vi "PROXY_display_messages_history.vi"(6 "station_in":T1, 8 "error_in":errorcluster, 9 "All Stations?":bool) -> (0 "error_out":errorcluster)   [LabVIEW 2020]
uses:
  STATION/station.ctl
  FGV/DIAGNOSTICS_message_history_buffer/PROXY_DIAGNOSTICS_message_history_buffer_all_info.ctl
  _misc/DIAGNOSTICS_message_type.ctl
  FGV/DIAGNOSTICS_message_history_display/FGV_PROXY_DIAGNOSTICS_message_history_display.ctl
  FGV/DIAGNOSTICS_message_history_buffer/FGV_PROXY_DIAGNOSTICS_message_history_buffer.ctl
  _misc/AULocalize/SubVIs/RegisterVI.vi
panel:
  in  "clear_messages":bool
  in  "STOP":bool
  in  "station_selector":u16(ring) caption="(ий)Station:" items=["(ий)Station 10", "(ий)Station 20", "(ий)Station 30", "(ий)Station 40", "(ий)Station 50", "(ий)Station 60", "(ий)Station 70", "(ий)Station 80", "(ий)Station 90", "(ий)Station 100", "(ий)Station 110", "(ий)Station 120", "(ий)Station 165", "(ий)ALL"]
  in  "refresh_messages":bool
  in  "messages_history_lbx":i32(listbox)
  # "Message History"
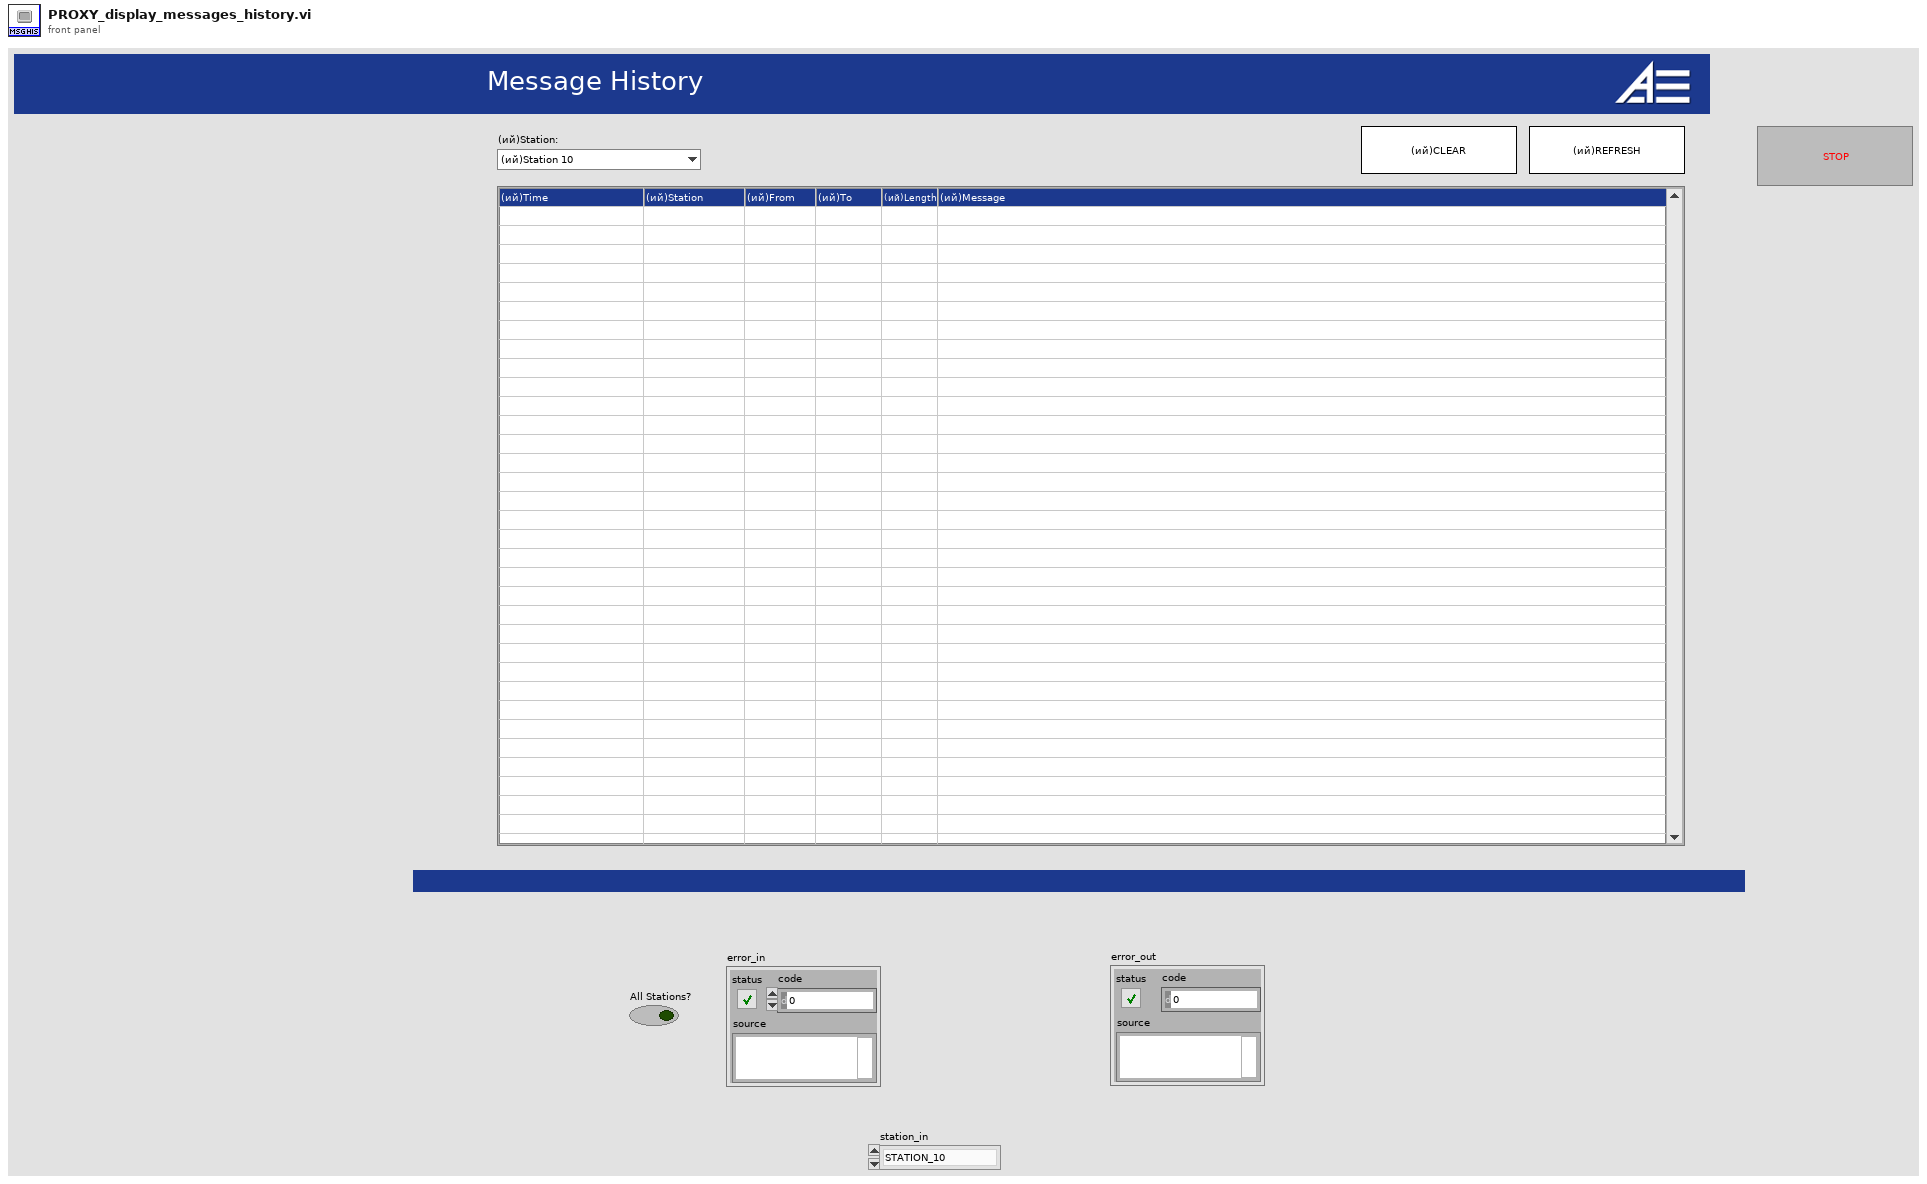
[diagram p1: front panel]
types:
  T1 = typedef "station.ctl" = enum16{"STATION_10", "STATION_20", "STATION_30", "STATION_40", "STATION_50", "STATION_60", "STATION_70", "STATION_80", "STATION_90", "STATION_100", "STATION_110", "STATION_120", "STATION_165", "MAIN"}
  T2 = typedef "FGV_PROXY_DIAGNOSTICS_message_history_display.ctl" = enum16{"initialize", "display_messages"}
  T3 = typedef "PROXY_DIAGNOSTICS_message_history_buffer_all_info.ctl" = cluster{"timestamp":timestamp, "station":T1, "message_type":T4, "message":string, "record":string[]}
  T4 = typedef "DIAGNOSTICS_message_type.ctl" = enum16{"TCP", "SQL"}
  T5 = typedef "FGV_PROXY_DIAGNOSTICS_message_history_buffer.ctl" = enum16{"initialize", "add_TCP_PLC_to_PC", "add_TCP_PC_to_PLC", "add_SQL_PC_to_DB", "add_SQL_transaction", "add_SQL_DB_to_PC", "get_station", "get_all", "clear_station", "clear_all", "save_log"}
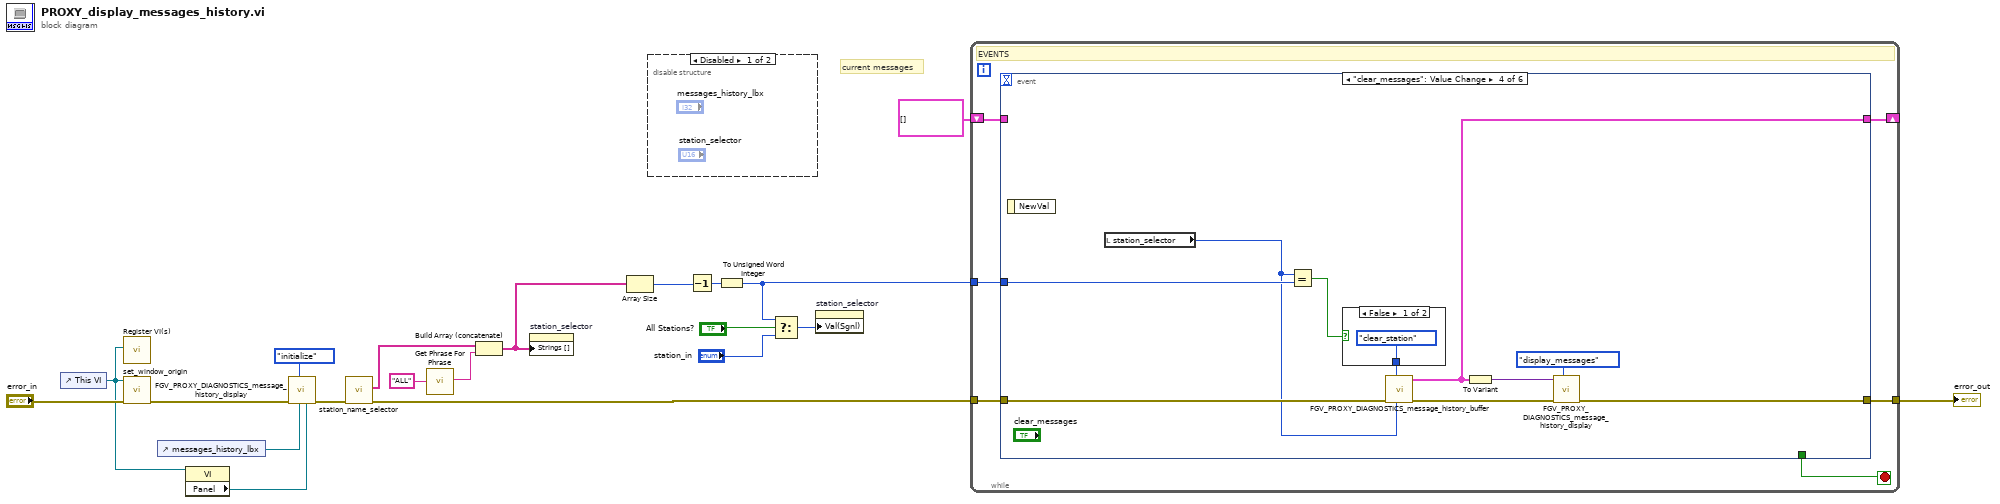
[diagram p0: block diagram]
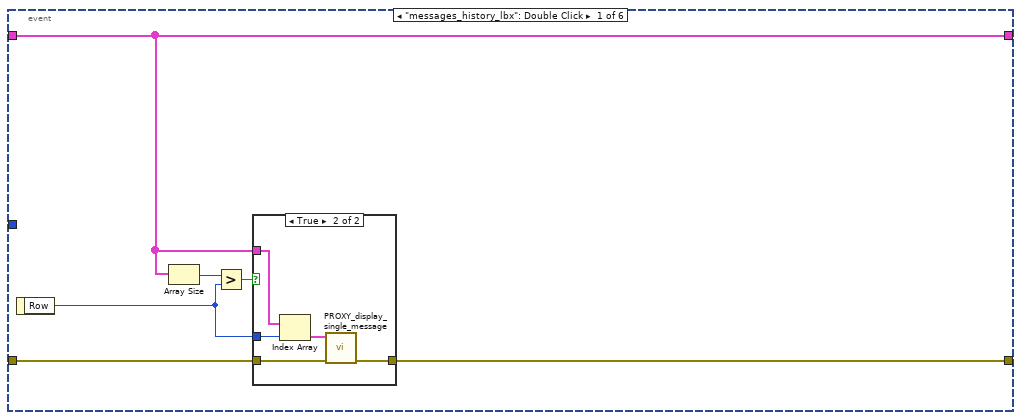
[diagram p3: hidden frame]
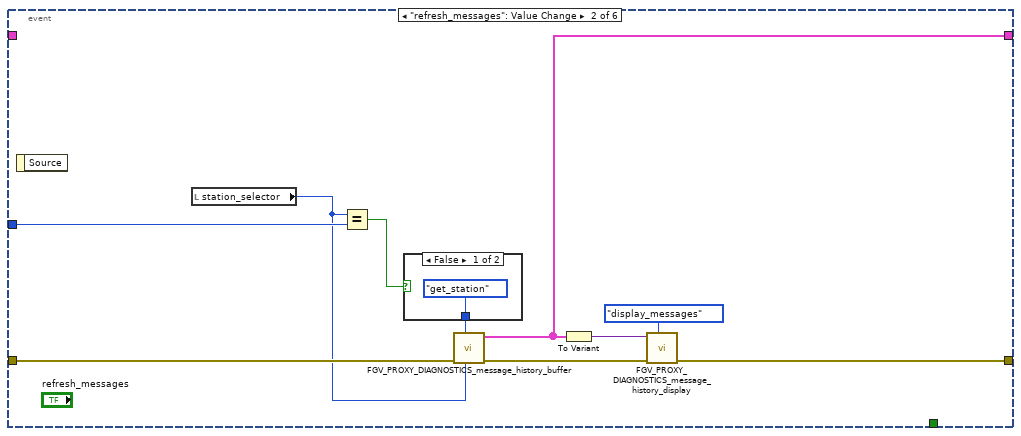
[diagram p5: hidden frame]
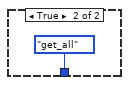
[diagram p6: hidden frame]
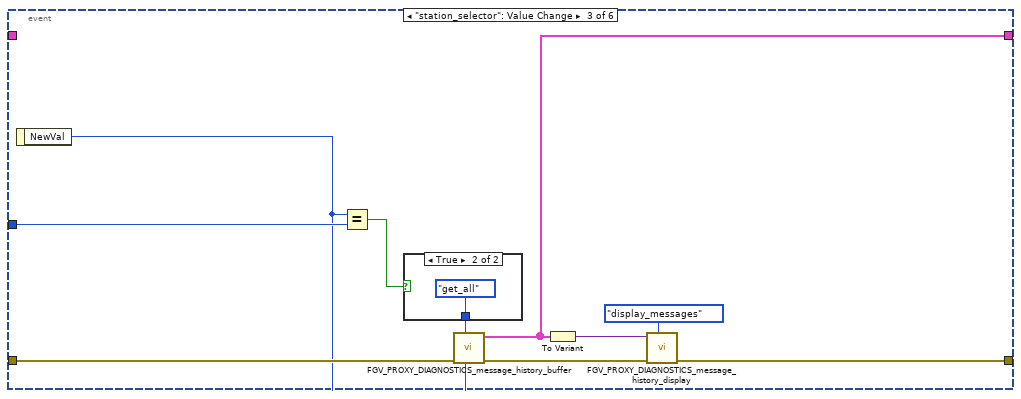
[diagram p7: hidden frame]
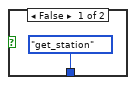
[diagram p8: hidden frame]
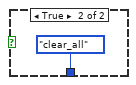
[diagram p9: hidden frame]
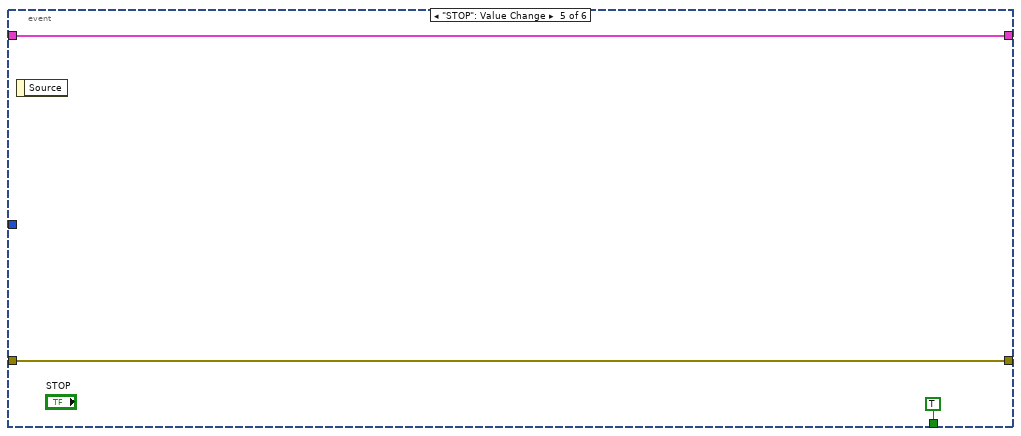
[diagram p10: hidden frame]
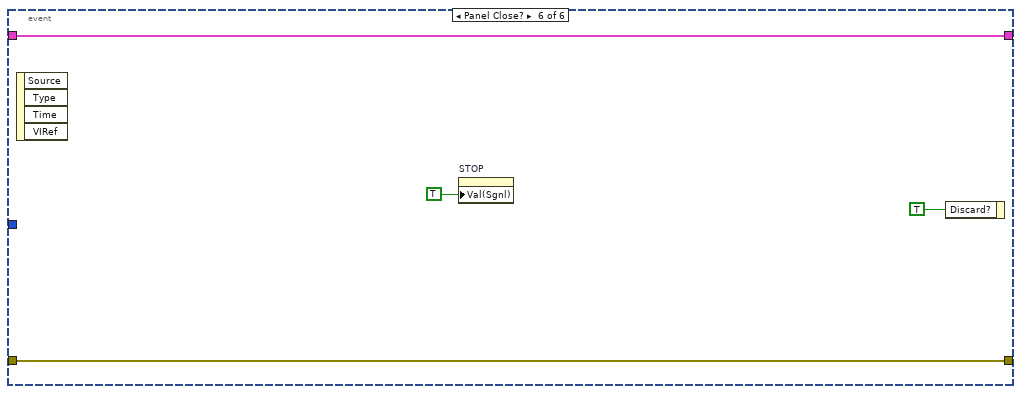
[diagram p11: hidden frame]
diagram:
  # "current messages"
  n1 = control-ref of="This VI"() -> (w3:refnum<vi>)
  n2 = call-poly "Register VI(s).vi"("VI Ref"=w3) -> ()  [unwired: 9 in, 2 out]
  n3 = call "set_window_origin.vi"("error_in"="error_in", "this_vi_reference"=w3) -> ("error_out"=w20:errorcluster)  [unwired: 9 in]
  n4 = control-ref of="messages_history_lbx"() -> (w18:refnum<vi>)
  n5 = property class="VI"(reference=w3) -> ("Panel"=w19:refnum<vi>)  [unwired: 1 in, 2 out]
  n6 = call "FGV_PROXY_DIAGNOSTICS_message_history_display.vi"("front_panel_reference"=w19, "SQL_listbox_reference"=w18, "options"=FGV_PROXY_DIAGNOSTICS_message_history_display."initialize", "error_in"=w20) -> ("error_out"=w15:errorcluster)  [unwired: 7 in]
  n7 = call "station_name_selector.vi"("error_in"=w15) -> ("error_out"=w12:errorcluster, "all_station_names"=w14:string[])  [unwired: 8 in, 1 out]
  n8 = call "Get Phrase For Phrase.vi"("Phrase"="ALL" ("ST30 name")) -> ("Phrase"=w1:string)  [unwired: 9 in, 1 out]
  n9 = Build Array (concatenate)(w14, w1) -> (w13:string[])
  n10 = property on="station_selector" class="Ring (strict)"("Strings []"=w13) -> ()  [unwired: 2 in, 2 out]
  n11 = Array Size(array=w13) -> (size(s)=w8:i32)
  n12 = disable-structure shown="Disabled" {
    frame Disabled {
    }
    frame Enabled {
    }
  }
  n13 = Decrement(x=w8) -> (x-1=w7:i32)
  n14 = To Unsigned Word Integer(number=w7) -> (unsigned 16bit integer=w6:u16)
  n15 = Select(t=w6, s="All Stations?", f="station_in") -> (s? t:f=w10:u16)
  n16 = property on="station_selector" class="Ring (strict)"("Val(Sgnl)"=w10) -> ()  [unwired: 2 in, 2 out]
  n17 = while {
    tunnel: [w26] -> w17
    tunnel: w12 -> [w24]
    tunnel: w6 -> [w23]
    shift-right: [w22] -> _
    shift-left: T3[] [] ("message_history") -> [w21]
    stop <- w25 stop-if-true
    # "EVENTS"
    n18 = event shown="[3] \"clear_messages\": Value Change" {
      selector: _ -> [_ _ _ _ _ _]
      dyn-events: _ -> [_ _ _ _ _ _]
      timeout: _ -> [_ _ _ _ _ _]
      tunnel: [_ _ _ _ TRUE _] -> w25
      tunnel: w24 -> [w32 w46 w58 w70 w77 w81]
      tunnel: [w31 w43 w54 w67 w77 w81] -> w26
      tunnel: w23 -> [_ w48 w60 w72 _ _]
      tunnel: [w30 w39 w51 w64 w75 w78] -> w22
      tunnel: w21 -> [w30 _ _ _ w75 w78]
      event "messages_history_lbx": Double Click {
        n19 = event-data() -> ("Row"=w28:i32)  [unwired: 1 in]
        n20 = Array Size(array=w30) -> (size(s)=w29:i32)
        n21 = Greater?(x=w29, y=w28) -> (0:w27:bool)
        n22 = case shown="True" w27 {
          tunnel: w32 -> [w33 w38]
          tunnel: [w33 w37] -> w31
          tunnel: w30 -> [_ w35]
          tunnel: w28 -> [_ w34]
          frame False {
          }
          frame True {
            n23 = Index Array(array=w35, index=w34) -> (element=w36:T3)
            n24 = call "PROXY_display_single_message.vi"("error_in"=w38, "message_history_buffer_element"=w36) -> ("error_out"=w37:errorcluster)  [unwired: 9 in]
          }
        }
      }
      event "refresh_messages": Value Change {
        n25 = event-data() -> ()  [unwired: 1 in, 1 out]
        n26 = local read "station_selector"() -> (w40:u16)
        n27 = Equal?(x=w40, y=w48) -> (x = y?=w45:bool)
        n28 = case shown="False" w45 {
          tunnel: [FGV_PROXY_DIAGNOSTICS_message_history_buffer."get_station" ("options") FGV_PROXY_DIAGNOSTICS_message_history_buffer."get_all" ("options")] -> w47
          frame False {
          }
          frame True {
          }
        }
        n29 = call "FGV_PROXY_DIAGNOSTICS_message_history_buffer.vi"("station"=w40, "options"=w47, "error_in"=w46) -> ("error_out"=w44:errorcluster, "message_history"=w39:T3[])  [unwired: 7 in]
        n30 = To Variant(anything=w39) -> (Variant=w42:variant)
        n31 = call "FGV_PROXY_DIAGNOSTICS_message_history_display.vi"("options"=FGV_PROXY_DIAGNOSTICS_message_history_display."display_messages", "error_in"=w44, "input"=w42) -> ("error_out"=w43:errorcluster)  [unwired: 8 in]
      }
      event "station_selector": Value Change {
        n32 = event-data() -> ("NewVal"=w56:u16)  [unwired: 1 in]
        n33 = Equal?(x=w56, y=w60) -> (x = y?=w57:bool)
        n34 = case shown="True" w57 {
          tunnel: [FGV_PROXY_DIAGNOSTICS_message_history_buffer."get_station" ("options") FGV_PROXY_DIAGNOSTICS_message_history_buffer."get_all" ("options")] -> w59
          frame False {
          }
          frame True {
          }
        }
        n35 = call "FGV_PROXY_DIAGNOSTICS_message_history_buffer.vi"("station"=w56, "options"=w59, "error_in"=w58) -> ("error_out"=w55:errorcluster, "message_history"=w51:T3[])  [unwired: 7 in]
        n36 = To Variant(anything=w51) -> (Variant=w53:variant)
        n37 = call "FGV_PROXY_DIAGNOSTICS_message_history_display.vi"("options"=FGV_PROXY_DIAGNOSTICS_message_history_display."display_messages", "error_in"=w55, "input"=w53) -> ("error_out"=w54:errorcluster)  [unwired: 8 in]
      }
      event "clear_messages": Value Change {
        n38 = event-data() -> ()  [unwired: 1 in, 1 out]
        n39 = local read "station_selector"() -> (w63:u16)
        n40 = Equal?(x=w63, y=w72) -> (x = y?=w69:bool)
        n41 = case shown="False" w69 {
          tunnel: [FGV_PROXY_DIAGNOSTICS_message_history_buffer."clear_station" ("options") FGV_PROXY_DIAGNOSTICS_message_history_buffer."clear_all" ("options")] -> w71
          frame False {
          }
          frame True {
          }
        }
        n42 = call "FGV_PROXY_DIAGNOSTICS_message_history_buffer.vi"("station"=w63, "options"=w71, "error_in"=w70) -> ("error_out"=w68:errorcluster, "message_history"=w64:T3[])  [unwired: 7 in]
        n43 = To Variant(anything=w64) -> (Variant=w66:variant)
        n44 = call "FGV_PROXY_DIAGNOSTICS_message_history_display.vi"("options"=FGV_PROXY_DIAGNOSTICS_message_history_display."display_messages", "error_in"=w68, "input"=w66) -> ("error_out"=w67:errorcluster)  [unwired: 8 in]
      }
      event "STOP": Value Change {
        n45 = event-data() -> ()  [unwired: 1 in, 1 out]
      }
      event Panel Close? {
        n46 = event-data() -> ()  [unwired: 1 in, 4 out]
        n47 = property on="STOP" class="Bool (strict)"("Val(Sgnl)"=TRUE ("Value (Signaling)")) -> ()  [unwired: 2 in, 2 out]
        n48 = event-data("Discard?"=TRUE) -> ()  [unwired: 1 in, 1 out]
      }
    }
  }
  "error_out" <- w17
